vi "Check Value Type.vi"(8 "error in (no error)":errorcluster, 11 "Column in":refnum<class "By-Value Column.lvclass">) -> (0 "error out":errorcluster, 3 "Column out":refnum<class "By-Value Column.lvclass">)   [LabVIEW 2020, in "Basic Columns.lvlib" / "By-Value Column.lvclass"]
uses:
  By-Value Column.lvclass
  Column Class/Column Parent.lvclass
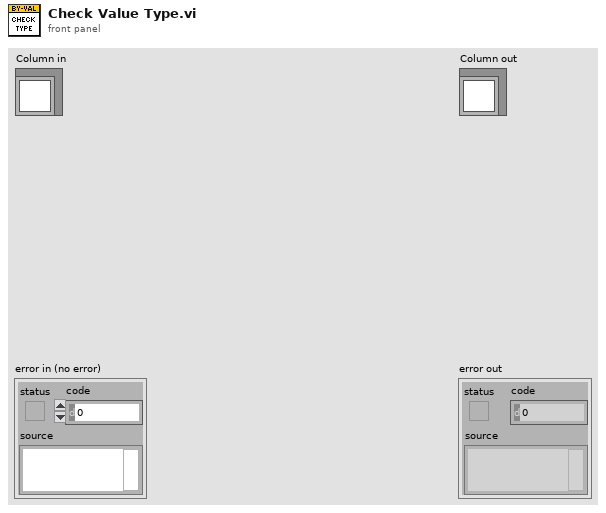
[diagram p1: front panel]
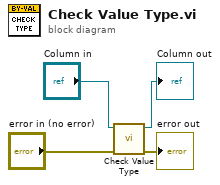
[diagram p0: block diagram]
diagram:
  n1 = call-parent "Check Value Type.vi"("error in (no error)"="error in (no error)", "Column in"="Column in") -> ("error out"=→"error out":errorcluster, "Column out"=→"Column out":refnum<class "By-Value Column.lvclass">)  [unwired: 8 in]
